vi "Create_Channel_Node_in XMLObject.vi"(8 "error in (no error)":errorcluster, 10 "Param Name-Value Array":T1(array[cluster]), 11 "Document Refnum IN":refnum<k20>) -> (0 "error out":errorcluster)   [LabVIEW 2012]
doc: "SciScan 1.2 160622"
uses:
  <vilib>/xml/NI_XML.lvlib
  <resource>/objmgr/DOMUserDefRef.rc
  GFG/GFG library.lvlib
panel:
  out "XML":string
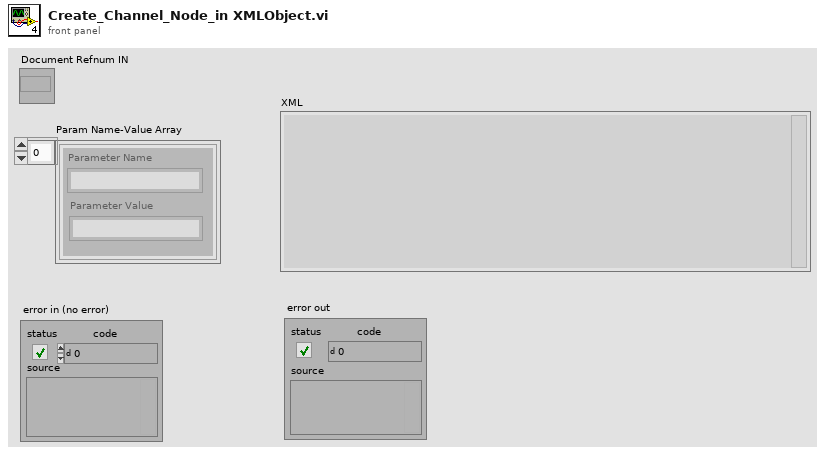
[diagram p1: front panel]
types:
  T1 = cluster{"Parameter Name":string, "Parameter Value":string}[]
  T2 = cluster{"Parameter Name":string, "Parameter Value":string}
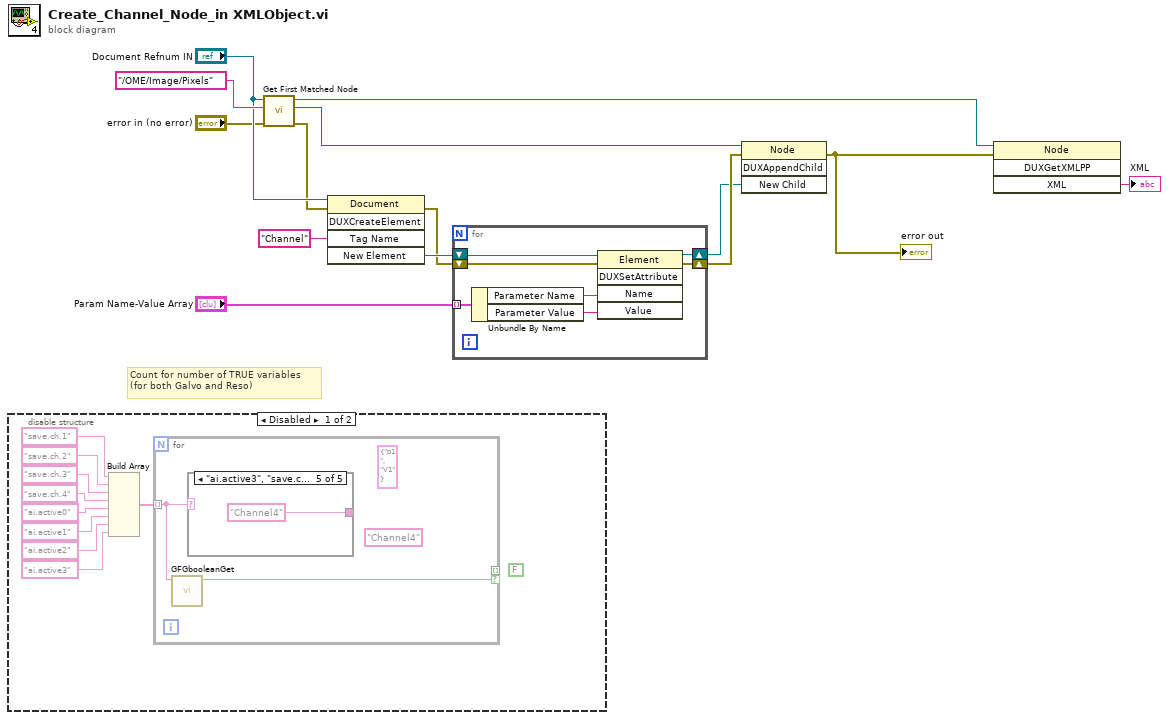
[diagram p0: block diagram]
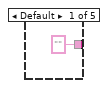
[diagram p2: hidden frame]
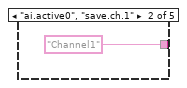
[diagram p3: hidden frame]
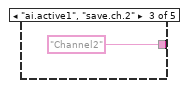
[diagram p4: hidden frame]
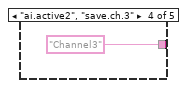
[diagram p5: hidden frame]
diagram:
  # "Count for number of TRUE variables\n(for both Galvo and Reso)"
  n1 = disable-structure shown="Disabled" {
    frame Disabled {
      (unwired) FALSE ("Boolean Value OUT")
      n2 = Build Array("save.ch.1" ("Variable Name in"), "save.ch.2" ("Variable Name in"), "save.ch.3" ("Variable Name in"), "save.ch.4" ("Variable Name in"), "ai.active0" ("Variable Name in"), "ai.active1" ("Variable Name in"), "ai.active2" ("Variable Name in"), "ai.active3" ("Variable Name in")) -> (w15:string[])
      n3 = for {
        tunnel: w15 -> [w24] mode=indexing
        tunnel: _ -> [_] mode=indexing if=w25
        (unwired) T2 {"Parameter Name"="p1", "Parameter Value"="V1"} ("Path-Value pairs")
        (unwired) "Channel4"
        n4 = call "GFGbooleanGet.vi"("Variable Name in"=w24) -> ("Boolean Value OUT"=w25:bool)  [unwired: 9 in, 1 out]
        n5 = case shown="\"ai.active3\", \"save.ch.4\"" w24 {
          tunnel: ["" "Channel1" "Channel2" "Channel3" "Channel4"] -> _
          frame Default {
          }
          frame "ai.active0", "save.ch.1" {
          }
          frame "ai.active1", "save.ch.2" {
          }
          frame "ai.active2", "save.ch.3" {
          }
          frame "ai.active3", "save.ch.4" {
          }
        }
      }
    }
    frame Enabled {
    }
  }
  n6 = call <vilib>:"Get First Matched Node.vi"("error in (no error)"="error in (no error)", "XPath expression"="/OME/Image/Pixels", "node in"="Document Refnum IN") -> ("error out"=w6:errorcluster, "node result"=w7:refnum<k20>, "node out"=w12:refnum<k20>)  [unwired: 6 in]
  n7 = invoke class="Document" method="DUXCreateElement"(reference="Document Refnum IN", error in=w6, "Tag Name"="Channel") -> (error out=w4:errorcluster, "New Element"=w9:refnum<k20>)  [unwired: 2 in, 3 out]
  n8 = for {
    tunnel: "Param Name-Value Array" -> [w33] mode=indexing
    shift-right: [w36] -> w8
    shift-left: w4 -> [w35]
    shift-right: [w34] -> w3
    shift-left: w9 -> [w37]
    n9 = Unbundle By Name(w33) -> ("Parameter Name"=w32:string, "Parameter Value"=w31:string)
    n10 = invoke class="Element" method="DUXSetAttribute"(reference=w37, error in=w35, "Name"=w32, "Value"=w31) -> (reference out=w34:refnum<k20>, error out=w36:errorcluster)  [unwired: 1 in, 3 out]
  }
  n11 = invoke class="Node" method="DUXAppendChild"(reference=w7, error in=w8, "New Child"=w3) -> (error out=w1:errorcluster)  [unwired: 1 in, 3 out]
  "error out" <- w1
  n12 = invoke class="Node" method="DUXGetXMLPP"(reference=w12, error in=w1) -> ("XML"=→"XML":string)  [unwired: 2 in, 3 out]
